vi "P4CMD Get Advanced Command Options.vi"(7 "advanced options in":variant, 8 "error in (no error)":errorcluster, 10 "command":T1 items=["GET", "CHECKOUT", "CHECKIN", "UNDOCHECKOUT", "ADD", "REMOVE", "COMPARE", "FILEHISTORY", "FILEPROPERTIES", "CONFIGOPTIONS"], 11 "source control reference in":T2) -> (0 "error out":errorcluster, 1 "dialog box cancelled?":bool, 2 "status message":string, 3 "source control reference out":T2, 5 "advanced options out":variant)   [LabVIEW 2017, in "NI_SCC_P4CMD.lvlib"]
uses:
  <vilib>/SourceControl/Providers/P4CMD/NI_SCC_P4CMD.lvlib
  <vilib>/SourceControl/sccapi/SCCAPI Refnum.ctl
  <vilib>/SourceControl/sccapi/SCCAPI Command.ctl
  <vilib>/SourceControl/Providers/P4CMD/P4CMD Advanced Options.ctl
  <vilib>/SourceControl/Providers/P4CMD/P4CMD Mgr Functions.ctl
  <vilib>/SourceControl/support/SCCSup Message Strings GLBL.vi
  <vilib>/SourceControl/sccapi/NI_SCC.lvlib
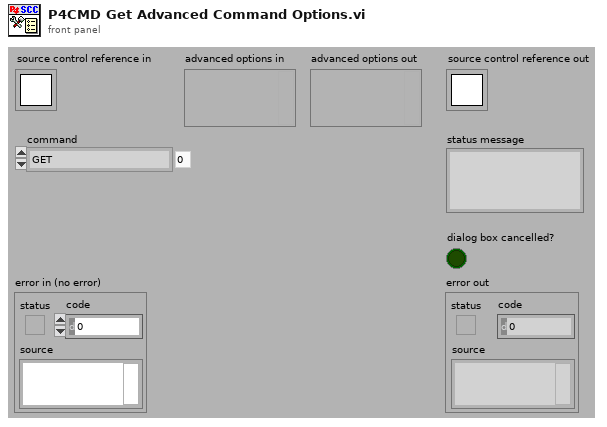
[diagram p1: front panel]
types:
  T1 = typedef "NI_SCC.lvlib/SCCAPI Command.ctl" = i32
  T2 = typedef "NI_SCC.lvlib/SCCAPI Refnum.ctl" = refnum<k1>
  T3 = typedef "NI_SCC_P4CMD.lvlib/P4CMD Advanced Options.ctl" = cluster{"lock files?":bool, "suppress dialogs?":bool}
  T4 = typedef "NI_SCC_P4CMD.lvlib/P4CMD Mgr Functions.ctl" = enum16{"Init", "Open", "Set Config Opts", "Initialized?", "IsRefValid?", "Get Config Opts", "Get Global Commands", "Close", "Uninit"}
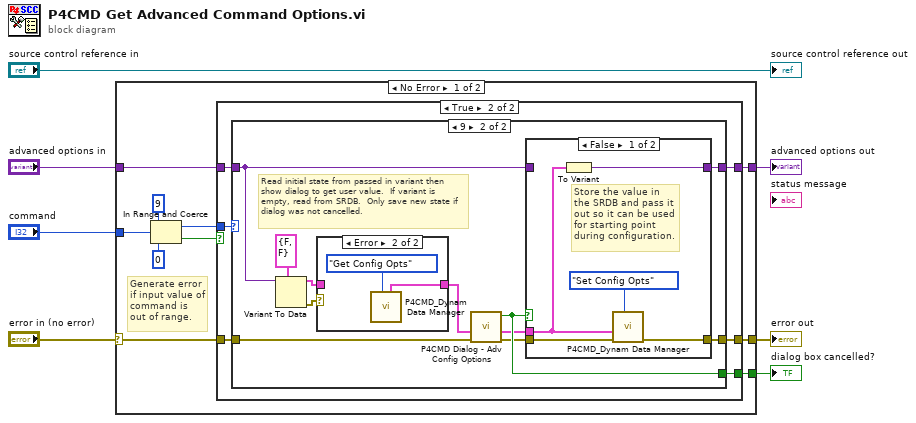
[diagram p0: block diagram]
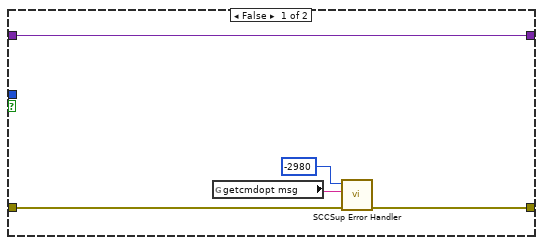
[diagram p2: hidden frame]
diagram:
  n1 = case shown="No Error" "error in (no error)" {
    selector: "error in (no error)" -> [w13 w53]
    tunnel: [w12 w53] -> w6
    tunnel: "command" -> [w15 _]
    tunnel: [w11 _] -> w3
    tunnel: "advanced options in" -> [w9 w52]
    tunnel: [w8 w52] -> w1
    frame No Error {
      # "Generate error if input value of command is out of range."
      n2 = In Range and Coerce(upper limit=9, x=w15, lower limit=0) -> (coerced(x)=w14:T1, In Range?=w10:bool)
      n3 = case shown="True" w10 {
        tunnel: w14 -> [_ w28]
        tunnel: w13 -> [w20 w27]
        tunnel: [w19 w26] -> w12
        tunnel: [_ w25] -> w11
        tunnel: w9 -> [w18 w24]
        tunnel: [w18 w23] -> w8
        frame False {
          n4 = global read "SCCSup Message Strings GLBL.vi" "getcmdopt msg"() -> (w21:string)
          n5 = call <vilib>:"SCCSup Error Handler.vi"("error in (no error)"=w20, "operation message"=w21, "scc error code"=-2980 ("error code")) -> ("error out"=w19:errorcluster)  [unwired: 8 in]
        }
        frame True {
          n6 = case shown="9" w28 {
            tunnel: w27 -> [w30 w34]
            tunnel: [w30 w41] -> w26
            tunnel: [_ w40] -> w25
            tunnel: w24 -> [w29 w36]
            tunnel: [w29 w37] -> w23
            frame Default {
            }
            frame 9 {
              # "Read initial state from passed in variant then show dialog to get user value.  If variant is empty, read from SRDB.  Only save new state if dialog was not cancelled."
              n7 = Variant To Data(type=T3 {"lock files?"=FALSE, "suppress dialogs?"=FALSE} ("adv cfg options out"), Variant=w36) -> (data=w32:T3, error out=w33:errorcluster)  [unwired: 1 in]
              n8 = case shown="Error" w33 {
                tunnel: w32 -> [w42 _]
                tunnel: [w42 w43] -> w31
                frame No Error {
                }
                frame Error {
                  n9 = call <vilib>:"P4CMD_Dynam Data Manager.vi"("function"=P4CMD_Mgr_Functions."Get Config Opts") -> ("adv cfg options out"=w43:T3)  [unwired: 5 in, 5 out]
                }
              }
              n10 = call <vilib>:"P4CMD Dialog - Adv Config Options.vi"("error in (no error)"=w34, "adv cfg options in"=w31) -> ("error out"=w39:errorcluster, "adv cfg  options out"=w38:T3, "cancelled?"=w40:bool)  [unwired: 7 in]
              n11 = case shown="False" w40 {
                tunnel: w39 -> [w48 w51]
                tunnel: [w47 w51] -> w41
                tunnel: w38 -> [w46 _]
                tunnel: w36 -> [_ w50]
                tunnel: [w45 w50] -> w37
                frame False {
                  # "Store the value in the SRDB and pass it out so it can be used for starting point during configuration."
                  n12 = To Variant(anything=w46) -> (Variant=w45:variant)
                  n13 = call <vilib>:"P4CMD_Dynam Data Manager.vi"("function"=P4CMD_Mgr_Functions."Set Config Opts", "error in (no error)"=w48, "adv cfg options in"=w46) -> ("error out"=w47:errorcluster)  [unwired: 3 in, 5 out]
                }
                frame True {
                }
              }
            }
          }
        }
      }
    }
    frame Error {
    }
  }
  "error out" <- w6
  "dialog box cancelled?" <- w3
  "advanced options out" <- w1
  "source control reference out" <- "source control reference in"
